vi "Save SerialParameters (SubVI).vi"(6 "FlashBaud":refnum<vi>, 7 "appended path":path, 9 "CmdBaud":refnum<vi>, 10 "COM Port":refnum<vi>, 11 "Path in":refnum<vi>) -> ()   [LabVIEW 2017]
uses:
  <vilib>/Utility/config.llb/Write Key (String).vi
  <vilib>/Utility/config.llb/NI_LVConfig.lvlib
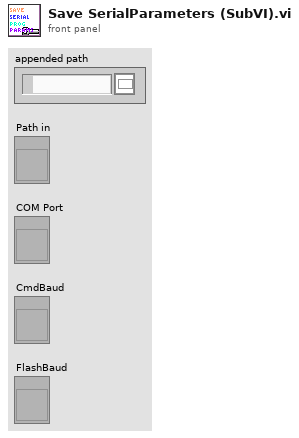
[diagram p1: front panel]
types:
  T1 = typedef "NI_LVConfig.lvlib/Config Data RefNum.ctl" = refnum<k1>
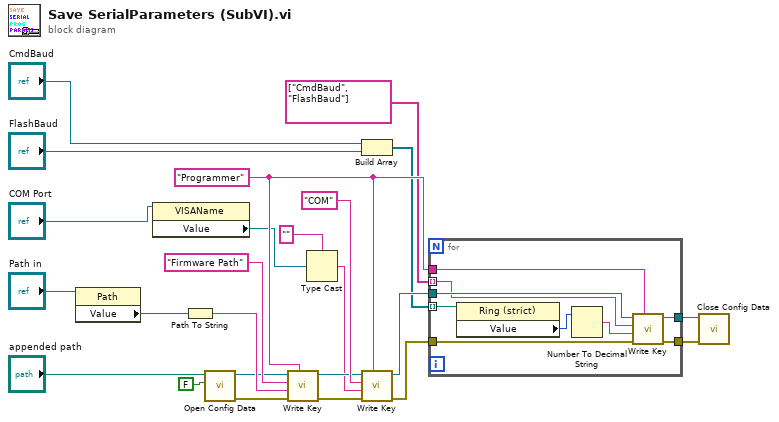
[diagram p0: block diagram]
diagram:
  w20 = "Programmer" ("section")
  n1 = property on="Property Node" class="Path"(reference="Path in") -> ("Value"=w10:path)  [unwired: 1 in, 2 out]
  n2 = property on="Property Node" class="VISAName"(reference="COM Port") -> ("Value"=w6:refnum<visa-resource-name>)  [unwired: 1 in, 2 out]
  n3 = Path To String(path=w10) -> (string=w9:string)
  n4 = call <vilib>:"Open Config Data.vi"("create file if necessary (T)"=FALSE, "configuration file path"="appended path") -> ("error out"=w7:errorcluster, "refnum"=w8:T1)  [unwired: 1 in, 7 out]
  n5 = call-poly <vilib>:"Write Key.vi"("section"=w20, "error in (no error)"=w7, "value"=w9, "key"="Firmware Path", "refnum"=w8) -> ("error out"=w17:errorcluster, "refnum out"=w15:T1)  [unwired: 1 in, 4 out]
  n6 = Type Cast(type="", x=w6) -> (*(type *) &x=w13:string)
  n7 = Build Array("CmdBaud", "FlashBaud") -> (w2:refnum<vi>[])
  n8 = call-poly <vilib>:"Write Key.vi"("section"=w20, "error in (no error)"=w17, "value"=w13, "key"="COM", "refnum"=w15) -> ("error out"=w16:errorcluster, "refnum out"=w14:T1)  [unwired: 1 in, 4 out]
  n9 = for {
    tunnel: w20 -> [w32]
    tunnel: w16 -> [w30]
    tunnel: [w28] -> w12
    tunnel: w14 -> [w29]
    tunnel: [w33] -> w24
    tunnel: w2 -> [w26] mode=indexing
    tunnel: string[] ["CmdBaud", "FlashBaud"] -> [w25] mode=indexing
    n10 = property on="Property Node" class="Ring (strict)"(reference=w26) -> ("Value"=w27:u32)  [unwired: 1 in, 2 out]
    n11 = Number To Decimal String(number=w27) -> (decimal integer string=w31:string)  [unwired: 1 in]
    n12 = call-poly <vilib>:"Write Key.vi"("section"=w32, "error in (no error)"=w30, "value"=w31, "key"=w25, "refnum"=w29) -> ("error out"=w28:errorcluster, "refnum out"=w33:T1)  [unwired: 1 in, 4 out]
  }
  n13 = call <vilib>:"Close Config Data.vi"("error in (no error)"=w12, "refnum"=w24) -> ()  [unwired: 1 in, 9 out]
